vi "Update Temp Setpoint.vi"(8 "error in (no error)":errorcluster, 10 "Setpoint (C)":dbl, 11 "Chamber Controller in":refnum<class "Chamber Controller.lvclass">) -> (0 "error out":errorcluster, 3 "Chamber Controller out":refnum<class "Chamber Controller.lvclass">)   [LabVIEW 2020, in "Chamber Controller.lvlib" / "Chamber Controller.lvclass"]
uses:
  Chamber Controller.lvclass
  Chamber Controller.lvclass/Chamber Controller.ctl
  _Abstract Classes/Abstract Chamber/Abstract Chamber.lvclass
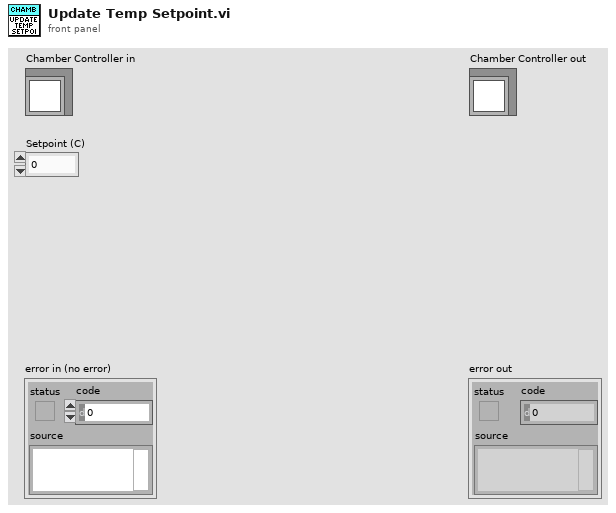
[diagram p1: front panel]
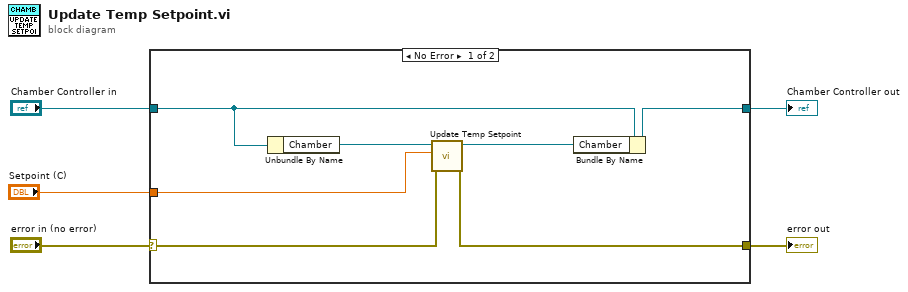
[diagram p0: block diagram]
diagram:
  n1 = case shown="No Error" "error in (no error)" {
    selector: "error in (no error)" -> [w8 w14]
    tunnel: [w7 w14] -> w4
    tunnel: [w10 w13] -> w2
    tunnel: "Chamber Controller in" -> [w12 w13]
    tunnel: "Setpoint (C)" -> [w6 _]
    frame No Error {
      n2 = Unbundle By Name(w12) -> ("Chamber"=w11:refnum<class "Abstract Chamber.lvclass">)
      n3 = call-dynamic "Update Temp Setpoint.vi"("error in (no error)"=w8, "Setpoint (C)"=w6, "Abstract Chamber in"=w11) -> ("error out"=w7:errorcluster, "Abstract Chamber out"=w9:refnum<class "Abstract Chamber.lvclass">)  [unwired: 7 in]
      n4 = Bundle By Name(cluster=w12, "Chamber"=w9) -> (w10:refnum<class "Chamber Controller.lvclass">)
    }
    frame Error {
    }
  }
  "error out" <- w4
  "Chamber Controller out" <- w2
